vi "Connect.vi"(8 "error in (no error)":errorcluster, 11 "Smart_Eye_Pro_Driver in":refnum<class "SmartEyeProDriver.lvclass">) -> (0 "error out":errorcluster, 3 "Smart_Eye_Pro_Driver out":refnum<class "SmartEyeProDriver.lvclass">)   [LabVIEW 2020, in "SmartEyeProDriver.lvclass"]
uses:
  SmartEyeProDriver.lvclass
  SmartEyeProDriver.lvclass/SmartEyeProDriver.ctl
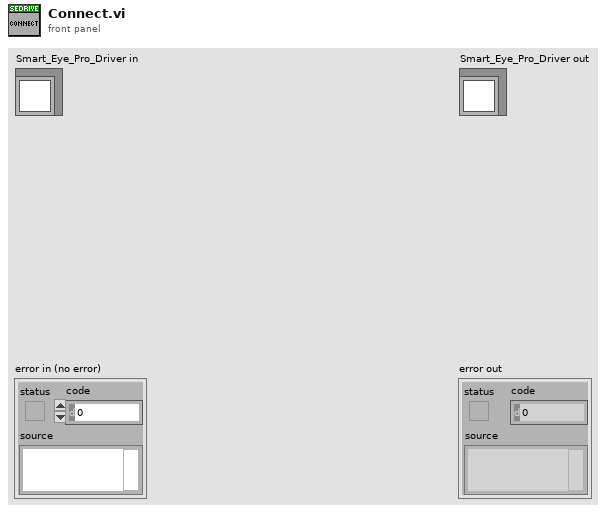
[diagram p1: front panel]
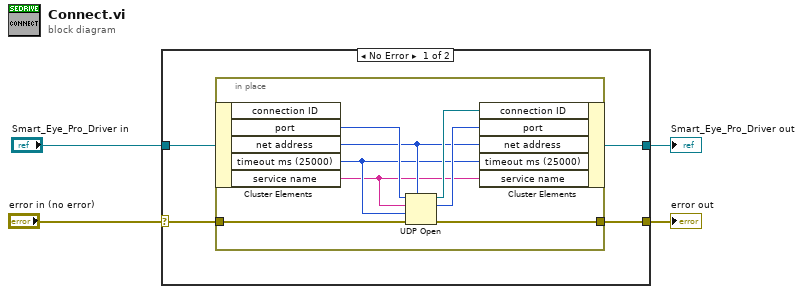
[diagram p0: block diagram]
diagram:
  n1 = case shown="No Error" "error in (no error)" {
    selector: "error in (no error)" -> [w7 w18]
    tunnel: [w6 w18] -> w3
    tunnel: [w5 w17] -> w1
    tunnel: "Smart_Eye_Pro_Driver in" -> [w8 w17]
    frame No Error {
      n2 = in-place {
        in-place-border: w7 -> [w16]
        in-place-border: [w15] -> w6
        n3 = in-place-cluster #1(w8) -> ("port"=w13:u16, "net address"=w11:u32, "timeout ms (25000)"=w10:i32, "service name"=w9:string)  [unwired: 1 out]
        n4 = UDP Open(7:w11, 8:w16, 9:w10, 10:w9, 11:w13) -> (port=w14:refnum<k16>, 0:w15:errorcluster, 2:w12:u16)
        n5 = in-place-cluster #1("connection ID"=w14, "port"=w12, "net address"=w11, "timeout ms (25000)"=w10, "service name"=w9) -> (w5:refnum<class "SmartEyeProDriver.lvclass">)
      }
    }
    frame Error {
    }
  }
  "error out" <- w3
  "Smart_Eye_Pro_Driver out" <- w1
